vi "Array comparision.vi"(11 "Array":dbl[][](array[numeric])) -> (3 "initialized array":dbl[][](array[numeric]))   [LabVIEW 2020]
doc: "If the last value in array is equal to speed of light, entire plot and array memory must be erased - for the proton cannot get past the lightspeed barier."
panel:
  # "SubVi to clear array after end of animation"
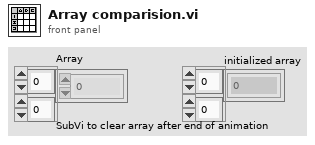
[diagram p1: front panel]
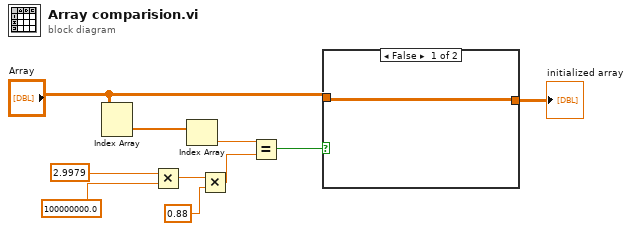
[diagram p0: block diagram]
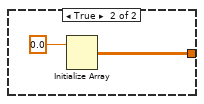
[diagram p2: hidden frame]
diagram:
  n1 = Index Array(array="Array") -> (element=w2:dbl[])  [unwired: 2 in]
  n2 = Multiply(x=2.9979, y=100000000.0) -> (x*y=w5:dbl)
  n3 = Index Array(array=w2) -> (element=w1:dbl)  [unwired: 1 in]
  n4 = Multiply(x=w5, y=0.88) -> (x*y=w3:dbl)
  n5 = Equal?(x=w1, y=w3) -> (x = y?=w8:bool)
  n6 = case shown="False" w8 {
    tunnel: [w11 w12] -> w9
    tunnel: "Array" -> [w11 _]
    frame False {
    }
    frame True {
      n7 = Initialize Array(0.0 ("element")) -> (w12:dbl[][])  [unwired: 2 in]
    }
  }
  "initialized array" <- w9
